vi "query_cmd.vi"(8 "error in (no error)":errorcluster, 10 "Command":string, 11 "connection ID":refnum<k5>) -> (0 "error out":errorcluster, 2 "Response":string, 3 "connection ID out":refnum<k5>)   [LabVIEW 2018]
panel:
  out "bytes written":i32
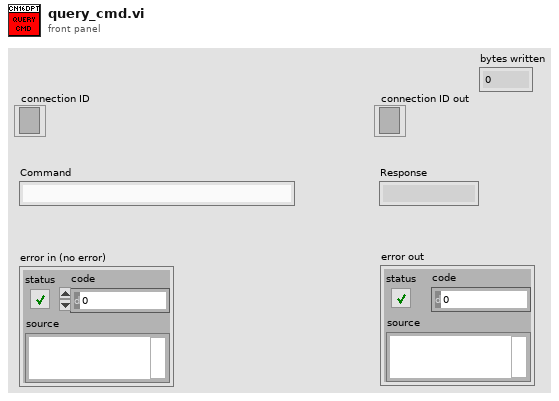
[diagram p1: front panel]
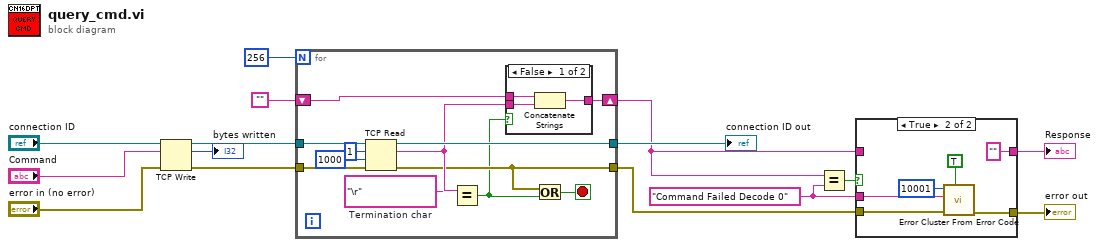
[diagram p0: block diagram]
diagram:
  w10 = "Command Failed Decode 0" ("y")
  n1 = TCP Write(connection ID="connection ID", data in="Command", error in (no error)="error in (no error)") -> (connection ID out=w4:refnum<k5>, bytes written=→"bytes written":i32, error out=w13:errorcluster)  [unwired: 1 in]
  n2 = for {
    N: 256 -> [_]
    tunnel: [w25] -> w6
    tunnel: w13 -> [w27]
    tunnel: [w19] -> w11
    tunnel: w4 -> [w24]
    shift-right: [w22] -> w2
    shift-left: "" -> [w21]
    stop <- w20 stop-if-true
    w16 = "\r"  # Termination char
    n3 = TCP Read(connection ID=w24, bytes to read=u32 1 ("byte count"), error in (no error)=w27, 9:1000 ("timeout ms (25000)")) -> (connection ID out=w25:refnum<k5>, data out=w23:string, error out=w19:errorcluster)  [unwired: 1 in]
    n4 = Equal?(x=w23, y=w16) -> (x = y?=w18:bool)
    n5 = case shown="False" w18 {
      tunnel: w23 -> [w30 _]
      tunnel: [w29 w31] -> w22
      tunnel: w21 -> [w28 w31]
      frame False {
        n6 = Concatenate Strings(w28, w30) -> (w29:string)
      }
      frame True {
      }
    }
    n7 = Or(x=w19, y=w18) -> (x .or. y?=w20:bool)
  }
  "connection ID out" <- w6
  n8 = Equal?(x=w2, y=w10) -> (x = y?=w12:bool)
  n9 = case shown="True" w12 {
    tunnel: w11 -> [w32 w37]
    tunnel: w10 -> [_ w36]
    tunnel: w2 -> [w33 _]
    tunnel: [w32 w35] -> w9
    tunnel: [w33 "" ("read buffer")] -> w8
    frame False {
    }
    frame True {
      n10 = call <vilib>:"Error Cluster From Error Code.vi"("show call chain? (False)"=TRUE, "error in (no error)"=w37, "error message (\"\")"=w36, "error code (0)"=10001) -> ("error out"=w35:errorcluster)  [unwired: 5 in]
    }
  }
  "Response" <- w8
  "error out" <- w9
